vi "Initialize.vi"(8 "error in":errorcluster, 10 "shared resources":refnum<class "Shared Resources.lvclass">, 11 "Rx Execution Unit Implementation in":refnum<class "Rx Execution Unit.lvclass">) -> (0 "error out":errorcluster, 3 "Rx Execution Unit Implementation out":refnum<class "Rx Execution Unit.lvclass">)   [LabVIEW 2020, in "Ballard MIL-STD-1553 Engine.lvlib" / "Implementation.lvlib" / "Rx Execution Unit.lvclass"]
uses:
  Rx Execution Unit.lvclass
  Execution Unit/Execution Unit.lvclass
  Custom Device/Custom Device.lvlib
  Shared Resources/Shared Resources.lvclass
  C:/Users/nitest/Desktop/Git 2020/niveristand-aim-milStd1553-custom-device/Source/Custom Device Support/Engine/Implementation/Execution Unit/Execution Unit.lvclass
  Interfaces/Shared Resources/Shared Resources.lvclass
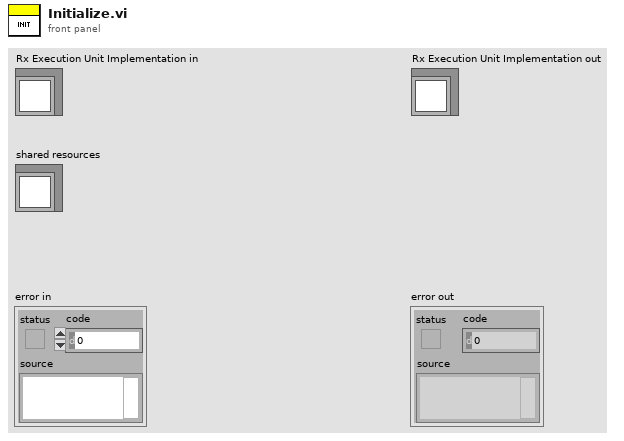
[diagram p1: front panel]
types:
  T1 = typedef "1553 Channel.ctl" = cluster{"HW channel":u16, "terminal addresses":T2[], "terminal names":string[], "acyclic frame names":string[], "messages":T3[]}
  T2 = typedef "Address.ctl" = u16
  T3 = typedef "Message Definition.ctl" = cluster{"name":string, "message type":T4, "endpoint Tx":T5, "endpoint Rx":T5, "create timestamp channel":bool, "mode code":u16, "number of words":u16, "parameters":cluster{"name":string, "default value":dbl, "unit":string, "parameter definition":T6}[]}
  T4 = typedef "Message Type.ctl" = string
  T5 = typedef "Terminal Endpoint.ctl" = cluster{"terminal address":T2, "subaddress":T2}
  T6 = typedef "Parameter Definition.ctl" = cluster{"start index":i32, "size (bits)":i32, "encoding":enum16{"BNR", "BCD", "Discrete"}, "signed":bool, "multiplier":dbl, "offset":dbl}
  T7 = typedef "Ballard MIL-STD-1553 Engine.lvlib/Implementation.lvlib/Execution Unit.lvclass/1553 Channel Handles.ctl" = cluster{"messages":T8[], "error count channel refs":T11, "terminal status channels":T10[]}
  T8 = typedef "Ballard MIL-STD-1553 Engine.lvlib/Implementation.lvlib/Execution Unit.lvclass/Message Handles.ctl" = cluster{"parameters":T9[], "timestamps":T10[], "Tx status handles":T10[], "Rx status handles":T10[]}
  T9 = typedef "Ballard MIL-STD-1553 Engine.lvlib/Implementation.lvlib/Execution Unit.lvclass/Parameter Handles.ctl" = cluster{"Tx channel handle":T10, "RxRT channel handle":T10, "RxBC channel handle":T10}
  T10 = typedef "Custom Device API.lvlib/Custom Device Item Ref.ctl" = u64
  T11 = typedef "Error Count Channel Refs.ctl" = cluster{"general protocol":T10, "improper number of words":T10, "Manchester":T10, "monitor":T10, "parity":T10, "unconfigured frames":T10, "word":T10, "wrong sync":T10}
  T12 = typedef "Ballard MIL-STD-1553 Engine.lvlib/Custom Device.lvlib/Hardware Handles.ctl" = cluster{"core handle":u64, "core reader handle":u64, "channel handles":u64[]}
  T13 = typedef "Rx Read Info.ctl" = cluster{"transfer handle":u64, "terminal address":u16}
  T14 = typedef "Ballard MIL-STD-1553 Engine.lvlib/Implementation.lvlib/Rx Execution Unit.lvclass/Status Terminal Lookup Data.ctl" = cluster{"value index":i32, "remote terminal handle":u64, "terminal address":u64}
  T15 = typedef "Map of Messages to Value Indexes.ctl" = map{T16, T17}
  T16 = typedef "Message Map Key.ctl" = cluster{"HW channel":u16, "terminal address":u16, "subaddress":u16, "mode code":u16}
  T17 = typedef "Ballard MIL-STD-1553 Engine.lvlib/Implementation.lvlib/Rx Execution Unit.lvclass/Message Map Value.ctl" = cluster{"value indexes":i32[], "message":T3, "Tx status count":i32, "Rx status count":i32}
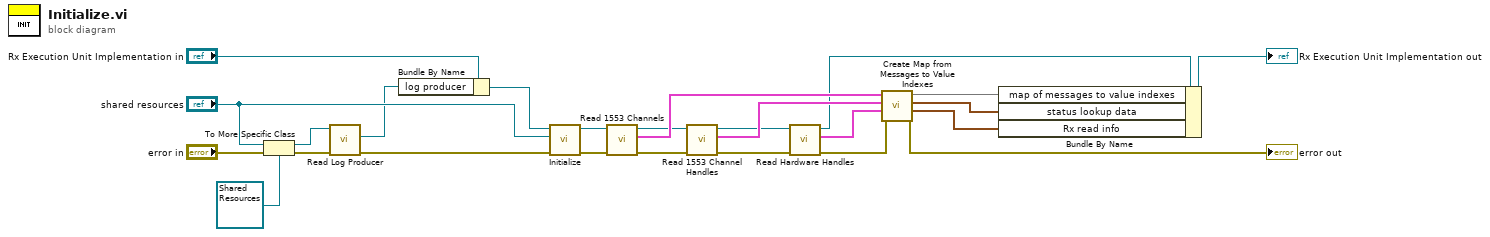
[diagram p0: block diagram]
diagram:
  n1 = To More Specific Class(target class=refnum<class "Shared Resources.lvclass"> refnum ("Shared Resources in"), reference="shared resources", error in="error in") -> (specific class reference=w12:refnum<class "Shared Resources.lvclass">, error out=w14:errorcluster)
  n2 = call-dynamic "Read Log Producer.vi"("error in (no error)"=w14, "Shared Resources in"=w12) -> ("error out"=w17:errorcluster, "Communication Bus Template Interfaces:Implementation.lvlib:Word Logging.lvlib:Log Producer.lvclass"=w11:refnum<class "Log Producer.lvclass">)  [unwired: 7 in, 1 out]
  n3 = Bundle By Name(cluster="Rx Execution Unit Implementation in", "log producer"=w11) -> (w9:refnum<class "Rx Execution Unit.lvclass">)
  n4 = call-parent "Initialize.vi"("error in"=w17, "shared resources"="shared resources", "Execution Unit Implementation in"=w9) -> ("error out"=w24:errorcluster, "Execution Unit Implementation out"=w25:refnum<class "Rx Execution Unit.lvclass">)  [unwired: 7 in]
  n5 = call "Read 1553 Channels.vi"("error in"=w24, "Execution Unit in"=w25) -> ("error out"=w19:errorcluster, "1553 channels"=w22:T1[], "Execution Unit out"=w20:refnum<class "Rx Execution Unit.lvclass">)  [unwired: 7 in]
  n6 = call "Read 1553 Channel Handles.vi"("error in"=w19, "Execution Unit in"=w20) -> ("error out"=w8:errorcluster, "1553 channel handles"=w18:T7[], "Execution Unit out"=w7:refnum<class "Rx Execution Unit.lvclass">)  [unwired: 7 in]
  n7 = call "Read Hardware Handles.vi"("error in"=w8, "Execution Unit in"=w7) -> ("error out"=w3:errorcluster, "hardware handles"=w1:T12, "Execution Unit out"=w6:refnum<class "Rx Execution Unit.lvclass">)  [unwired: 7 in]
  n8 = call "Create Map from Messages to Value Indexes.vi"("error in"=w3, "hardware handles"=w1, "1553 channel handles"=w18, "1553 channels"=w22) -> ("error out"=→"error out":errorcluster, "Rx read info"=w2:T13[], "status lookup data"=w5:T14[], "map from messages to value indexes"=w21:T15)  [unwired: 4 in]
  n9 = Bundle By Name(cluster=w6, "map of messages to value indexes"=w21, "status lookup data"=w5, "Rx read info"=w2) -> (→"Rx Execution Unit Implementation out":refnum<class "Rx Execution Unit.lvclass">)
